vi "DC Motor Direction Control.vi"() -> ()   [LabVIEW 2015]
doc: "This example performs writes and reads on a serial port, as directed by the user. You can press the Write and Read buttons, and change the Read Count, while the example is running.\n\nThe parameters set for the serial port must match the parameters of the connected instrument or device. In this example, the Read Count parameter specifies the number of bytes that the serial port reads. If there were more bytes at the port than the specified number, those bytes would not be read. If there were less bytes at the port than the specified number, you would receive a timeout error.\n\nThis example expands upon the flow control options for XON and XOFF, allowing the user to choose those control characters. Also, the user can enable or disable a termination character. Some devices require a termination character in order to identify the end of command strings. Some devices send a termination character to signify the end of data to be read. This example shows how you can end the Read operation once a termination character is detected in the buffer and/or append a termination character at the end of the Write data."
uses:
  <vilib>/Instr/_visa.llb/VISA Configure Serial Port (Instr).vi
panel:
  in  "Stop":bool
  in  "Stop Motor":bool
  in  "Anti\nclockwise":bool
  in  "Clocckwise":bool
  out "Executed Commands":string
  in  "Start  Program":bool
  in  "Arduino COM port":refnum<visa-resource-name>="COM1"
  # "DC Motor Direction Control using NI LabVIEW"
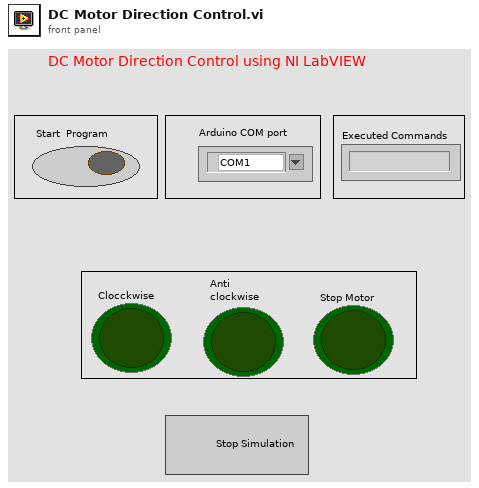
[diagram p1: front panel]
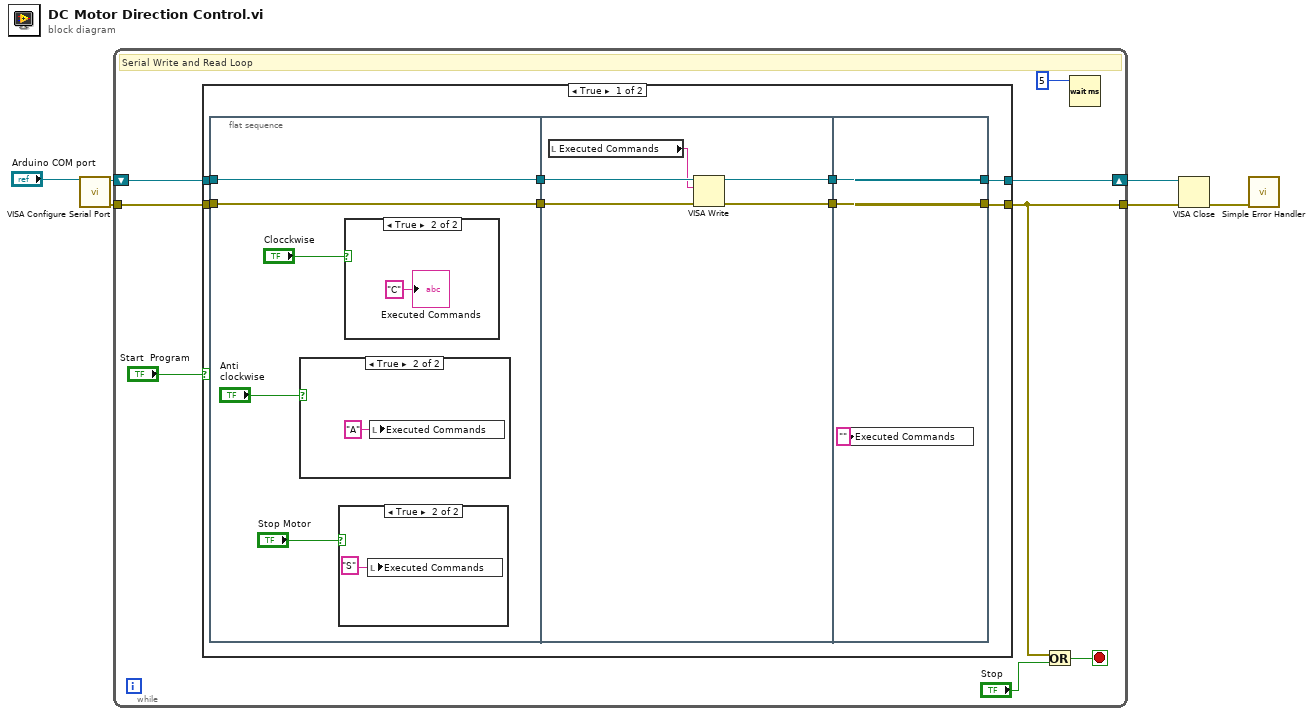
[diagram p0: block diagram]
diagram:
  n1 = call-poly "VISA Configure Serial Port"("VISA resource name"="Arduino COM port") -> ("VISA resource name out"=w3:refnum<visa-resource-name>, "error out"=w2:errorcluster)  [unwired: 9 in, 4 out]
  n2 = while {
    shift-right: [w14] -> w4
    shift-left: w3 -> [w11]
    tunnel: w2 -> [w10]
    tunnel: [w12] -> w5
    stop <- w8 stop-if-true
    # "Serial Write and Read Loop"
    n3 = case shown="True" "Start  Program" {
      tunnel: [w20 w40] -> w14
      tunnel: w11 -> [w22 w40]
      tunnel: [w19 w39] -> w12
      tunnel: w10 -> [w21 w39]
      frame True {
        n4 = flat-sequence {
          tunnel: w21 -> [w26]
          tunnel: w22 -> [w27]
          tunnel: [w27] -> w18
          tunnel: [w26] -> w17
          tunnel: w18 -> [w35]
          tunnel: w17 -> [w34]
          tunnel: [w33] -> w16
          tunnel: [w32] -> w15
          tunnel: [w37] -> w19
          tunnel: [w38] -> w20
          tunnel: w16 -> [w38]
          tunnel: w15 -> [w37]
          frame #0 {
            n5 = case shown="True" "Anti\nclockwise" {
              frame False {
              }
              frame True {
                n6 = local write "Executed Commands"("A") -> ()
              }
            }
            n7 = case shown="True" "Stop Motor" {
              frame False {
              }
              frame True {
                n8 = local write "Executed Commands"("S" ("Command Box")) -> ()
              }
            }
            n9 = case shown="True" "Clocckwise" {
              frame False {
              }
              frame True {
                "Executed Commands" <- "C" ("Command Box")
              }
            }
          }
          frame #1 {
            n10 = local read "Executed Commands"() -> (w31:string)
            n11 = VISA Write(VISA resource name=w35, write buffer=w31, error in (no error)=w34) -> (VISA resource name out=w33:refnum<visa-resource-name>, error out=w32:errorcluster)  [unwired: 1 out]
          }
          frame #2 {
            n12 = local write "Executed Commands"("" ("Command Box")) -> ()
          }
        }
      }
      frame False {
      }
    }
    n13 = Or(x=w12, y="Stop") -> (x .or. y?=w8:bool)
    n14 = Wait (ms)(milliseconds to wait=u32 5) -> ()  [unwired: 1 out]
  }
  n15 = VISA Close(VISA resource name=w4, error in (no error)=w5) -> (error out=w6:errorcluster)
  n16 = call <vilib>:"Simple Error Handler.vi"("error in (no error)"=w6) -> ()  [unwired: 1 in, 8 out]
